vi "kDSAtest.vi"() -> ()   [LabVIEW 2010, in "kevLib2011.lvlib"]
uses:
  kevLib2011.lvlib
  DSACntVariables.ctl
panel:
  out "Imag":dbl[](array[numeric])
  out "Re":dbl[](array[numeric])
  out "Waveform Chart 3":dbl(graph)
  in  "DSA Control Variables":T1={"High Freq"=200.1, "Sample Time"=0.001, "Low Freq"=10.1, "Num Data Points"=10, "Num Periods"=10, "Settling Time"=0.1}
  out "excitation signal":dbl
  out "Frequencies":dbl[](array[numeric])
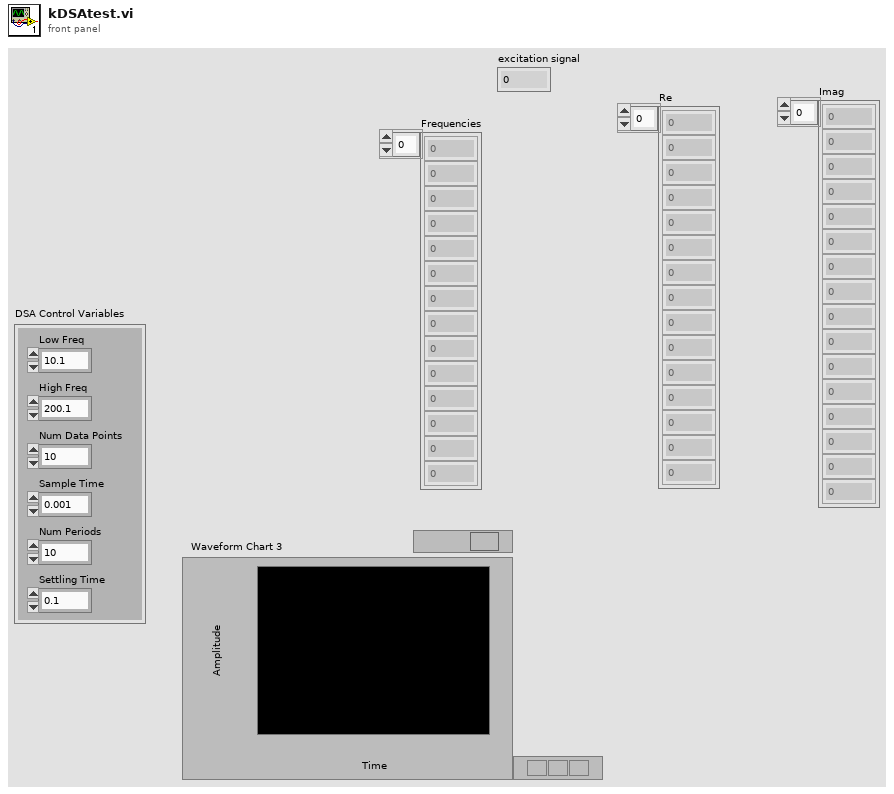
[diagram p1: front panel]
types:
  T1 = typedef "kevLib2011.lvlib/DSACntVariables.ctl" = cluster{"High Freq":dbl, "Sample Time":dbl, "Low Freq":dbl, "Num Data Points":i32, "Num Periods":i32, "Settling Time":dbl}
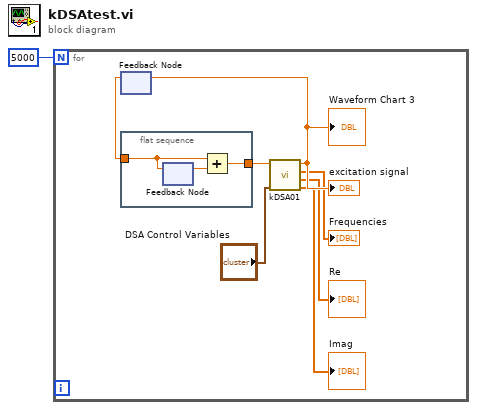
[diagram p0: block diagram]
diagram:
  n1 = for {
    N: 5000 -> [_]
    n2 = feedback #1() -> (w8:dbl)  [unwired: 1 in]
    n3 = flat-sequence {
      tunnel: w8 -> [w10]
      tunnel: [w9] -> w7
      frame #0 {
        n4 = feedback #2() -> (w11:dbl)  [unwired: 1 in]
        n5 = feedback-in #2(w10) -> ()
        n6 = Add(x=w10, y=w11) -> (x+y=w9:dbl)
      }
    }
    n7 = call "kDSA01.vi"("DSA Control Variables"="DSA Control Variables", "Sensor Reading"=w7) -> ("Imag"=→"Imag":dbl[], "Re"=→"Re":dbl[], "Frequencies"=→"Frequencies":dbl[], "excitation signal"=w5:dbl)  [unwired: 6 in]
    "excitation signal" <- w5
    "Waveform Chart 3" <- w5
    n8 = feedback-in #1(w5) -> ()
  }
